vi "Timestamp to String.vi"(1 "Time Stamp":timestamp) -> (0 "date/time string":string)   [LabVIEW 2020, in "Caraya.lvlib" / "Basic Test Manager.lvclass"]
uses:
  Basic Test Manager.lvclass
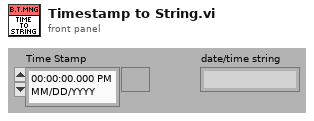
[diagram p1: front panel]
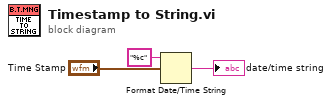
[diagram p0: block diagram]
diagram:
  n1 = Format Date/Time String(time format string (%c)="%c", seconds (now)="Time Stamp") -> (date/time string=→"date/time string":string)  [unwired: 1 in]
